vi "Update Disabled Deselect.vi"(8 "error in (no error)":errorcluster, 10 "Disabled Deselect Button":T1(ring), 11 "Lite Tools View in":refnum<class "Lite Tools View.lvclass">) -> (0 "error out":errorcluster, 3 "Lite Tools View out":refnum<class "Lite Tools View.lvclass">)   [LabVIEW 2020, in "Lite Tools View.lvlib" / "Lite Tools View.lvclass"]
uses:
  Lite Tools View.lvclass
  Lite Tools View.lvclass/Lite Tools View.ctl
panel:
  # "NOTICE -- YOU MUST LEAVE THIS NOTICE IN PLACE.\n\nCopyright (c) 2017, LIANG LIU Shawn.Liu.cn@gmail.com\nAll rights reserved.\n\nRedistribution and use in source and binary forms, with or without modification, are permitted provided that the following conditions are met:\n-Redistributions of source code must retain the above copyright notice, this list of conditions and the following disclaimer.\n-Redistributions in binary form must reproduce the above copyright notice, this list of conditions and the following disclaimer in the documentation and/or other materials provided with the distribution.\n-Neither the name of the eLp nor the names of its contributors may be used to endorse or promote products derived from this software without specific prior written permission.\n\nTHIS SOFTWARE IS PROVIDED BY THE COPYRIGHT HOLDERS AND CONTRIBUTORS \"AS IS\" AND ANY EXPRESS OR IMPLIED WARRANTIES, INCLUDING, BUT NOT LIMITED TO, THE IMPLIED WARRANTIES OF MERCHANTABILITY AND FITNESS FOR A PARTICULAR PURPOSE ARE DISCLAIMED. IN NO EVENT SHALL THE COPYRIGHT HOLDER OR CONTRIBUTORS BE LIABLE FOR ANY DIRECT, INDIRECT, INCIDENTAL, SPECIAL, EXEMPLARY, OR CONSEQUENTIAL DAMAGES (INCLUDING, BUT NOT LIMITED TO, PROCUREMENT OF SUBSTITUTE GOODS OR SERVICES; LOSS OF USE, DATA, OR PROFITS; OR BUSINESS INTERRUPTION) HOWEVER CAUSED AND ON ANY THEORY OF LIABILITY, WHETHER IN CONTRACT, STRICT LIABILITY, OR TORT (INCLUDING NEGLIGENCE OR OTHERWISE) ARISING IN ANY WAY OUT OF THE USE OF THIS SOFTWARE, EVEN IF ADVISED OF THE POSSIBILITY OF SUCH DAMAGE."
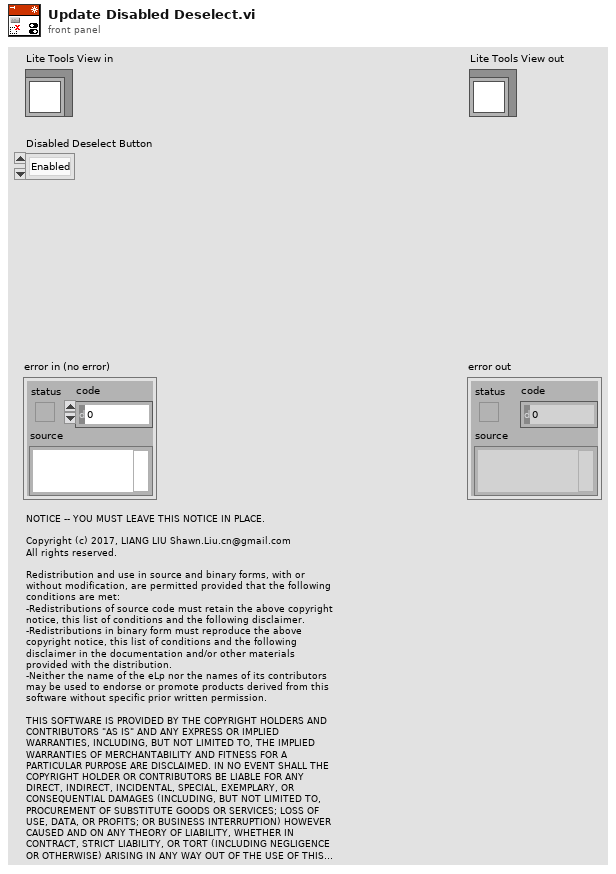
[diagram p1: front panel]
types:
  T1 = enum8{"Enabled", "Disabled", "Disabled and Grayed Out"}
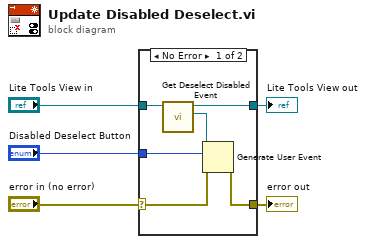
[diagram p0: block diagram]
diagram:
  n1 = case shown="No Error" "error in (no error)" {
    selector: "error in (no error)" -> [w8 w13]
    tunnel: "Lite Tools View in" -> [w11 w12]
    tunnel: [w10 w12] -> w1
    tunnel: "Disabled Deselect Button" -> [w9 _]
    tunnel: [w7 w13] -> w2
    frame No Error {
      n2 = call "Get Deselect Disabled Event.vi"("Lite Tools View in"=w11) -> ("Deselect Disabled Event"=w6:refnum<user-event>, "Lite Tools View out"=w10:refnum<class "Lite Tools View.lvclass">)  [unwired: 9 in]
      n3 = Generate User Event(user event=w6, event data cluster=w9, error in=w8) -> (error out=w7:errorcluster)  [unwired: 1 in, 1 out]
    }
    frame Error {
    }
  }
  "error out" <- w2
  "Lite Tools View out" <- w1
